vi "WILT Create Valve Array.vi"(11 "Water Valves Cluster":T1) -> (2 "Station Number":i32, 3 "Water Valve Array":bool[](array[boolean]), 5 "Valve Found!!":bool)   [LabVIEW 2016]
uses:
  Type Definitions/WILT Water Valve Cluster.ctl
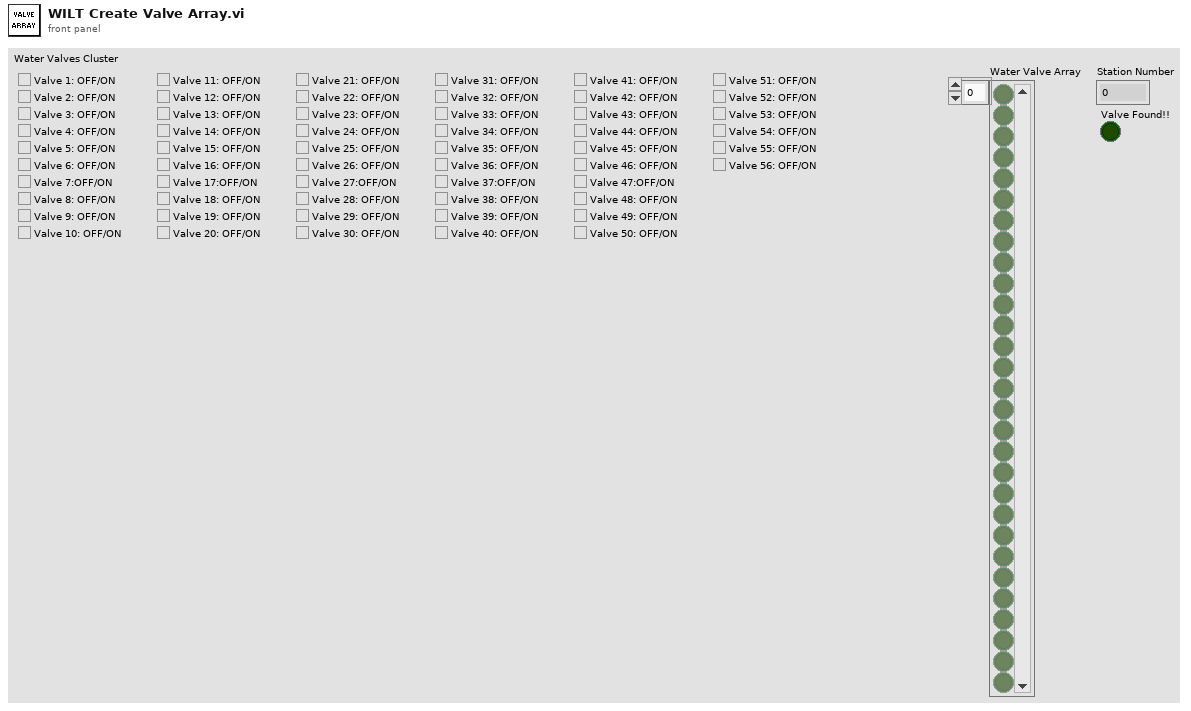
[diagram p1: front panel]
types:
  T1 = typedef "WILT Water Valve Cluster.ctl" = cluster{"Valve 1":bool, "Valve 2":bool, "Valve 3":bool, "Valve 4":bool, "Valve 5":bool, "Valve 6":bool, "Valve 7":bool, "Valve 8":bool, "Valve 9":bool, "Valve 10":bool, "Valve 11":bool, "Valve 12":bool, "Valve 13":bool, "Valve 14":bool, "Valve 15":bool, "Valve 16":bool, "Valve 17":bool, "Valve 18":bool, "Valve 19":bool, "Valve 20":bool, "Valve 21":bool, "Valve 22":bool, "Valve 23":bool, "Valve 24":bool, "Valve 25":bool, "Valve 26":bool, "Valve 27":bool, "Valve 28":bool, "Valve 29":bool, "Valve 30":bool, "Valve 31":bool, "Valve 32":bool, "Valve 33":bool, "Valve 34":bool, "Valve 35":bool, "Valve 36":bool, "Valve 37":bool, "Valve 38":bool, "Valve 39":bool, "Valve 40":bool, "Valve 41":bool, "Valve 42":bool, "Valve 43":bool, "Valve 44":bool, "Valve 45":bool, "Valve 46":bool, "Valve 47":bool, "Valve 48":bool, "Valve 49":bool, "Valve 50":bool, "Valve 51":bool, "Valve 52":bool, "Valve 53":bool, "Valve 54":bool, "Valve 55":bool, "Valve 56":bool}
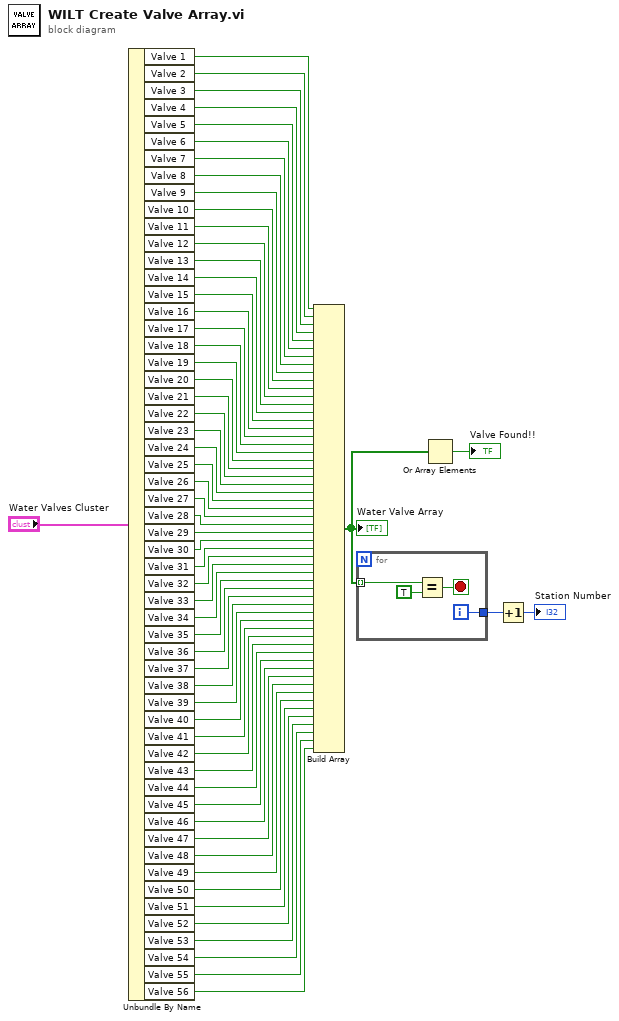
[diagram p0: block diagram]
diagram:
  n1 = Unbundle By Name("Water Valves Cluster") -> ("Valve 1"=w60:bool, "Valve 2"=w59:bool, "Valve 3"=w58:bool, "Valve 4"=w57:bool, "Valve 5"=w56:bool, "Valve 6"=w55:bool, "Valve 7"=w54:bool, "Valve 8"=w53:bool, "Valve 9"=w52:bool, "Valve 10"=w51:bool, "Valve 11"=w50:bool, "Valve 12"=w49:bool, "Valve 13"=w48:bool, "Valve 14"=w47:bool, "Valve 15"=w46:bool, "Valve 16"=w45:bool, "Valve 17"=w44:bool, "Valve 18"=w43:bool, "Valve 19"=w42:bool, "Valve 20"=w41:bool, "Valve 21"=w40:bool, "Valve 22"=w39:bool, "Valve 23"=w38:bool, "Valve 24"=w37:bool, "Valve 25"=w36:bool, "Valve 26"=w35:bool, "Valve 27"=w34:bool, "Valve 28"=w33:bool, "Valve 29"=w32:bool, "Valve 30"=w31:bool, "Valve 31"=w30:bool, "Valve 32"=w29:bool, "Valve 33"=w28:bool, "Valve 34"=w27:bool, "Valve 35"=w26:bool, "Valve 36"=w25:bool, "Valve 37"=w24:bool, "Valve 38"=w23:bool, "Valve 39"=w22:bool, "Valve 40"=w21:bool, "Valve 41"=w20:bool, "Valve 42"=w19:bool, "Valve 43"=w18:bool, "Valve 44"=w17:bool, "Valve 45"=w16:bool, "Valve 46"=w15:bool, "Valve 47"=w14:bool, "Valve 48"=w13:bool, "Valve 49"=w12:bool, "Valve 50"=w11:bool, "Valve 51"=w10:bool, "Valve 52"=w9:bool, "Valve 53"=w8:bool, "Valve 54"=w7:bool, "Valve 55"=w6:bool, "Valve 56"=w5:bool)
  n2 = Build Array(w60, w59, w58, w57, w56, w55, w54, w53, w52, w51, w50, w49, w48, w47, w46, w45, w44, w43, w42, w41, w40, w39, w38, w37, w36, w35, w34, w33, w32, w31, w30, w29, w28, w27, w26, w25, w24, w23, w22, w21, w20, w19, w18, w17, w16, w15, w14, w13, w12, w11, w10, w9, w8, w7, w6, w5) -> (w2:bool[])
  "Water Valve Array" <- w2
  n3 = for {
    tunnel: w2 -> [w65] mode=indexing
    tunnel: [w62] -> w4
    i -> [w62]
    stop <- w63 stop-if-true
    n4 = Equal?(x=w65, y=TRUE) -> (x = y?=w63:bool)
  }
  n5 = Or Array Elements(Boolean array=w2) -> (logical OR=→"Valve Found!!":bool)
  n6 = Increment(x=w4) -> (x+1=→"Station Number":i32)
